vi "Msg To.vi"() -> (3 "Event Loop Msg out":refnum<class "Event Loop Msg.lvclass">)   [LabVIEW 2021, in "Event Loop.lvlib" / "Event Loop Msg.lvclass"]
uses:
  Event Loop Msg.lvclass
  Event Loop Msg.lvclass/Event Loop Msg.ctl
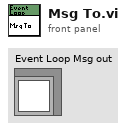
[diagram p1: front panel]
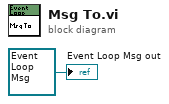
[diagram p0: block diagram]
diagram:
  "Event Loop Msg out" <- refnum<class "Event Loop Msg.lvclass"> refnum ("Event Loop Msg out")
